vi "Update Online List.vi"(8 "error in (no error)":errorcluster, 10 "Online List":string[](array[string]), 11 "Chat Window Interface in":refnum<class "Chat Window Interface.lvclass">) -> (0 "error out":errorcluster, 3 "Chat Window Interface out":refnum<class "Chat Window Interface.lvclass">)   [LabVIEW 2018, in "Chat Window Interface.lvlib" / "Chat Window Interface.lvclass"]
uses:
  Chat Window Interface.lvclass
  Chat Window Interface.lvclass/Chat Window Interface.ctl
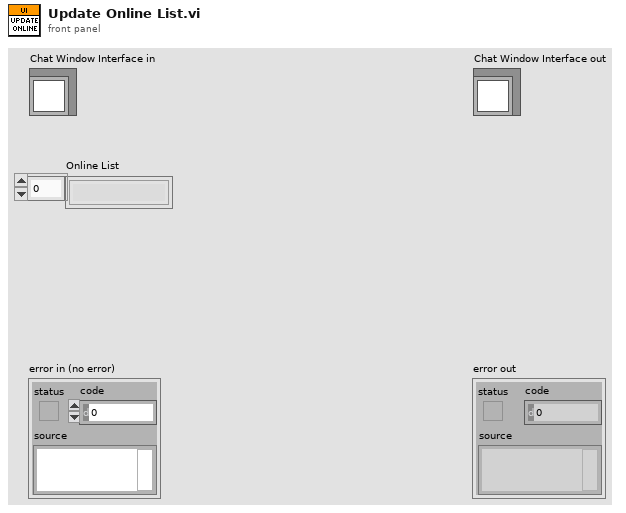
[diagram p1: front panel]
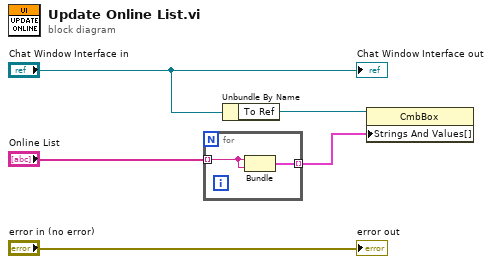
[diagram p0: block diagram]
diagram:
  n1 = for {
    tunnel: "Online List" -> [w6] mode=indexing
    tunnel: [w7] -> w1 mode=indexing
    n2 = Bundle("String"=w6, "String"=w6) -> (w7:cluster{"String":string, "String":string})  [unwired: 1 in]
  }
  n3 = Unbundle By Name("Chat Window Interface in") -> ("To Ref"=w3:refnum<vi>)
  n4 = property class="CmbBox"(reference=w3, "Strings And Values[]"=w1) -> ()  [unwired: 1 in, 2 out]
  "error out" <- "error in (no error)"
  "Chat Window Interface out" <- "Chat Window Interface in"
